vi "Log Scrolling Logic.vi"(8 "error in (no error)":errorcluster, 10 "System Log in":string, 11 "String in":refnum<vi>) -> (0 "error out":errorcluster, 2 "Scroll Postion Out":u32, 3 "System Log out":string caption="System Log")   [LabVIEW 2014, in "Testing UI 1.lvlib"]
uses:
  Testing UI 1.lvlib
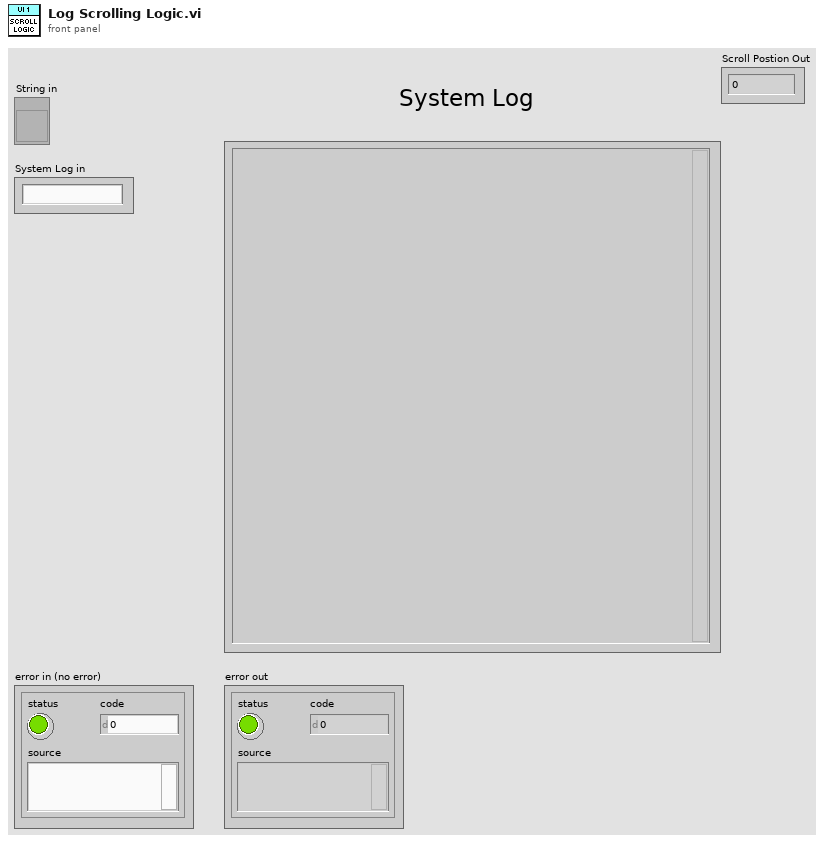
[diagram p1: front panel]
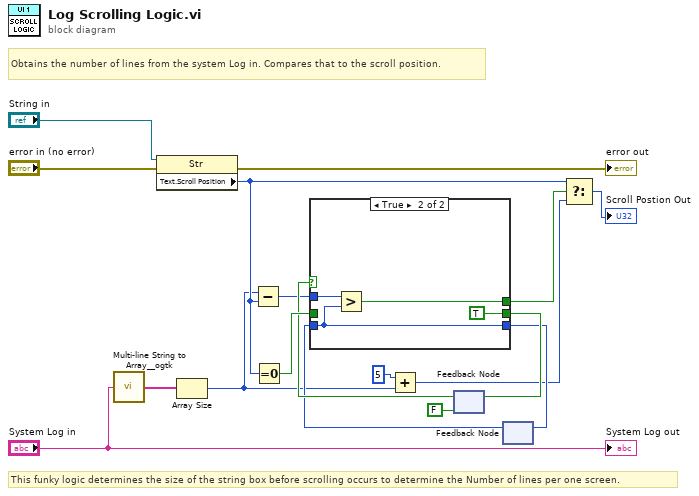
[diagram p0: block diagram]
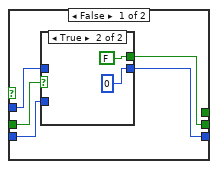
[diagram p2: hidden frame]
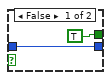
[diagram p3: hidden frame]
diagram:
  # "This funky logic determines the size of the string box before scrolling occurs to determine the Number of lines per one screen."
  # "Obtains the number of lines from the system Log in. Compares that to the scroll position."
  n1 = call <userlib>:"Multi-line String to Array__ogtk.vi"("string"="System Log in") -> ("lines"=w16:string[])
  n2 = property on="Property Node" class="Str"(reference="String in", error in="error in (no error)") -> (error out=→"error out":errorcluster, "Text.Scroll Position"=w14:u32)  [unwired: 1 out]
  n3 = Array Size(array=w16) -> (size(s)=w4:i32)
  n4 = Subtract(x=w4, y=w14) -> (x-y=w9:u32)
  n5 = Equal To 0?(x=w14) -> (x = 0?=w13:bool)
  n6 = Add(x=5, y=w4) -> (x+y=w2:i32)
  n7 = feedback #1(FALSE) -> (w12:bool)
  n8 = feedback #2() -> (w7:u32)  [unwired: 1 in]
  n9 = case shown="True" w12 {
    tunnel: w13 -> [w23 _]
    tunnel: [w22 TRUE] -> w11
    tunnel: [_ w30] -> w6
    tunnel: w7 -> [w21 w28]
    tunnel: [w20 w28] -> w8
    tunnel: w9 -> [w19 w29]
    frame False {
      n10 = case shown="True" w23 {
        tunnel: [TRUE FALSE] -> w22
        tunnel: w21 -> [_ _]
        tunnel: [w24 u32 0] -> w20
        tunnel: w19 -> [w24 _]
        frame False {
        }
        frame True {
        }
      }
    }
    frame True {
      n11 = Greater?(x=w29, y=w28) -> (0:w30:bool)
    }
  }
  n12 = feedback-in #1(w11) -> ()
  n13 = feedback-in #2(w8) -> ()
  n14 = Select(t=w14, s=w6, f=w2) -> (s? t:f=→"Scroll Postion Out":u32)
  "System Log out" <- "System Log in"
